vi "MainGUI.vi"() -> ()   [LabVIEW 2018]
uses:
  General/Controls/ScanType.ctl
  General/Controls/Vibratome Parameters.ctl
  General/Controls/Imaging Parameters.ctl
  General/Controls/Scan Direction.ctl
  General/type defines/Alazar parameters.ctl
  Hardware Mfg/AlazarTech SDK/Controls/General Trigger Settings.ctl
  Hardware Mfg/AlazarTech SDK/Controls/Trigger Engine Controls.ctl
  Hardware Mfg/AlazarTech SDK/Controls/Clock Controls.ctl
  Hardware Mfg/AlazarTech SDK/Controls/Alazar Device ID.ctl
  Hardware Mfg/AlazarTech SDK/Controls/Channel Input Controls.ctl
  Hardware Mfg/AlazarTech SDK/Controls/Alazar Acquisition Settings.ctl
  General/Controls/Optical Parameters.ctl
  General/Controls/Translation Stage Parameters.ctl
  Hardware Mfg/Thorlabs Translation Stages/Controls/Translation Stage Cluster.ctl
  General/Controls/Translation Stage Types.ctl
  General/Controls/Go Scan Actions.ctl
  General/Controls/Hardware control.ctl
  General/Controls/Queue Manager Actions.ctl
  General/Controls/MessagePacket.ctl
  General/Controls/QueueNames.ctl
  General/Controls/FGV Actions.ctl
  General/Controls/System Parameters.ctl
  Hardware Mfg/AlazarTech SDK/Controls/Alazar Engine Actions.ctl
  Hardware Mfg/Main Scan Processor Status.vi
  Hardware Mfg/Axsun Laser/Axsun action.ctl
panel:
  in  "Status":string
  in  "Quit":bool
  in  "Acquire":bool
  in  "Control Panel":T1(tab)
  in  "Optical Parameters":T2={"Obj. Focal Length [mm]"=45.0, "Scan Lens EFL[mm]"=59.5, "Tube Lens EFL[mm]"=205.0, "Galvo V Range (+/-)"=10.0, "Galvo Max Half Angle [Deg]"=19.0, "Max Galvo Range[%]"=0.0}
  in  "Galvo HW Parameters":T3={"Analog Out Channel"="GalvoCtrl/ao0,GalvoCtrl/ao1", "Min Voltage"=-10.0, "Max Voltage"=10.0, "Pixel Clock Source"="/GalvoCtrl/PFI0", "Sample Rate"=1000.0, "Line Clock Out Ch"="GalvoCtrl/port0/line0"}
  in  "Imaging Parameter":T4={"Raster Scan Direction"=enum."Uni Directional", "Pixel Dwell Time [Clock Cycles]"=1, "Flyback Time [Clock Cycles]"=200, "XY Center [um]"={"X"=1.0, "Y"=1.0}, "Pixel Step Size [um]"=2.5, "XY Image Size"=enum."2048 x 2048", "Custom"=TRUE, "Custom Size"={"X"=1200, "Y"=1200}, "Line Averages"=1} {"Line Averages" min=1 max=30 step=1; "Flyback Time [Clock Cycles]" max=1000 step=1; "Pixel Step Size [um]" min=0.0 max=10.0 step=0.01; "Custom Size"."Y" min=1 max=30 step=1; "Custom Size"."X" min=1 max=30 step=1; "XY Center [um]"."Y" min=1.0 max=30.0 step=1.0; "XY Center [um]"."X" min=1.0 max=30.0 step=1.0; "Pixel Dwell Time [Clock Cycles]" max=10 step=1}
  in  "Scan Type":T6
  in  "Hardware in":T7
  in  "Alazar parameters":T8={"Trigger Settings"={"General Trigger Settings"={"Trigger Operation"=0, "Coupling ID"=2, "Range ID"=2, "Delay"=0, "Timeout Ticks"=0, "Mode"=1, "Parameter"=1}, "Trigger Engine 1"={"Trigger Engine"=0, "Source"=2, "Slope"=1, "Level"=140}, "Trigger Engine 2"={"Trigger Engine"=1, "Source"=2, "Slope"=1, "Level"=2048}}, "Capture Clock"={"Sample Rate"=100, "Decimation"=0, "Source"=2, "Edge"=0}, "Device ID"={"System ID"=1, "Board ID"=1}, "Ch A Input Control"={"Channel"=1, "Coupling"=2, "Range"=10, "Impedance"=2}, "Ch B Input Control"={"Channel"=2, "Coupling"=2, "Range"=10, "Impedance"=2}, "Acq Settings"={"Window Type"=1, "Record Length"=1440, "Footer"=0, "Offset"=0, "Records Per Buffer"=1220, "Samples per record"=2048, "Records Count (Records/Acq)"=2147483647, "Output Format"=11}} {"Acq Settings"."Output Format" items=["Float Amp"=10, "Float Log"=11, "U16_LOG"=1, "U16_AMP2"=257]; "Acq Settings"."Window Type" items=["DSP_WINDOW_NONE", "DSP_WINDOW_HANNING", "DSP_WINDOW_HAMMING", "DSP_WINDOW_BLACKMAN", "DSP_WINDOW_BLACKMAN_HARRIS", "DSP_WINDOW_BARTLETT"]; "Acq Settings"."Footer" items=["FOOTER_NONE", "FOOTER_NPT"]; "Ch B Input Control"."Channel" items=["A"=1, "B"=2, "C"=4, "D"=8]; "Ch B Input Control"."Coupling" items=["AC"=1, "DC"=2]; "Ch B Input Control"."Range" items=["20 mV"=1, "40 mV"=2, "50 mV"=3, "80 mV"=4, "100 mV"=5, "200 mV"=6, "400 mV"=7, "500 mV"=8, "800 mV"=9, "1 V"=10, "1.25 V"=33, "2 V"=11, "4 V"=12, "5 V"=13, "8 V"=14, "10 V"=15, "20 V"=16]; "Ch B Input Control"."Impedance" items=["1 MOhm"=1, "50 Ohm"=2, ""=0]; "Ch A Input Control"."Channel" items=["A"=1, "B"=2, "C"=4, "D"=8]; "Ch A Input Control"."Coupling" items=["AC"=1, "DC"=2]; "Ch A Input Control"."Range" items=["20 mV"=1, "40 mV"=2, "50 mV"=3, "80 mV"=4, "100 mV"=5, "200 mV"=6, "400 mV"=7, "500 mV"=8, "800 mV"=9, "1 V"=10, "1.25 V"=33, "2 V"=11, "4 V"=12, "5 V"=13, "8 V"=14, "10 V"=15, "20 V"=16]; "Ch A Input Control"."Impedance" items=["1 MOhm"=1, "50 Ohm"=2, ""=0]; "Capture Clock"."Edge" items=["Rising", "Falling"]; "Capture Clock"."Source" items=["Internal"=1, "Fast External"=2, "Medium External"=3, "Slow External"=4, "External AC"=5, "External DC"=6, "External 10MHz"=7]; "Trigger Settings"."General Trigger Settings"."Trigger Operation" items=["J", "K", "J OR K", "J AND K", "J XOR K", "J AND NOT K", "NOT J AND K"]; "Trigger Settings"."General Trigger Settings"."Coupling ID" items=["AC"=1, "DC"=2]; "Trigger Settings"."General Trigger Settings"."Range ID" items=["5 V", "1 V", "TTL"]; "Trigger Settings"."Trigger Engine 1"."Trigger Engine" items=["J", "K"]; "Trigger Settings"."Trigger Engine 1"."Source" items=["A", "B", "External", "Disable", "C", "D"]; "Trigger Settings"."Trigger Engine 1"."Slope" items=["Positive"=1, "Negative"=2]; "Trigger Settings"."Trigger Engine 2"."Trigger Engine" items=["J", "K"]; "Trigger Settings"."Trigger Engine 2"."Source" items=["A", "B", "External", "Disable", "C", "D"]; "Trigger Settings"."Trigger Engine 2"."Slope" items=["Positive"=1, "Negative"=2]}
  in  "Vibratome":T15={"Z Bottom [mm]"=0.0, "Pre Cut Dwell [s]"=0.0, "Blade Frequency [RPM]"=0, "Slice Speed [mm/s]"=0.0, "Post Cut Dwell [s]"=0.0, "Ramp Time [s]"=0.0, "Start X [mm]"=0.0, "Start Y [mm]"=0.0, "Slice Length [mm]"=0.0, "Slice Axis"=enum."X Axis", "Controller VISA Ref"="COM4"}
  in  "Mosaic Paramter":T16
  in  "#pixels to save":u32=70
  in  "Start pixel for save":u32=70
  in  "Save?":bool
  in  "Center Galvos":bool
  in  "path":path=path "C:/Users/BOAS-USER/Documents/Data/0520/test"
  in  "#pixels to display":i32=500
  in  "Channel":u32(ring)=1 items=["A"=1, "B"=2, "A + B"=3, "C"=4, "A + C"=5, "A + B"=6, "D"=8, "A + D"=9, "B + D"=10, "C + D"=12, "A + B + C + D"=15]
  out "#C-lines":i32=1
  in  "Start pixel for display":i32=1
  out "Current Position":cluster{"X":dbl, "Y":dbl}
  out "Current state":T17
  in  "Table Stages":T18={"X Stage"={"Position"=0.0, "Is.Enabled?"=FALSE, "Is.Connected?"=FALSE, "Device SN"="45876539", "AccelerationMaximum"=20.0, "VelocityMaximum"=20.0, "Acceleration"=10.0, "Velocity"=10.0, "waitTimeout (ms)"=1000, "Model"=enum."Thorlabs LTS", "Is.Homed?"=FALSE}, "Y Stage"={"Position"=0.0, "Is.Enabled?"=FALSE, "Is.Connected?"=FALSE, "Device SN"="45875512", "AccelerationMaximum"=20.0, "VelocityMaximum"=20.0, "Acceleration"=10.0, "Velocity"=10.0, "waitTimeout (ms)"=1000, "Model"=enum."Thorlabs LTS", "Is.Homed?"=FALSE}, "Z Stage"={"Position"=0.0, "Is.Enabled?"=FALSE, "Is.Connected?"=FALSE, "Device SN"="49876924", "AccelerationMaximum"=8.0, "VelocityMaximum"=3.0, "Acceleration"=4.0, "Velocity"=2.0, "waitTimeout (ms)"=1000, "Model"=enum."Thorlabs MLJ", "Is.Homed?"=FALSE}}
  out "Image":T21(plugin-control)
  out "Control Class ID":u32[](array[numeric])
  out "Label Name":string[][](array[string])
  # "Image Settings"
  # "Optical Settings"
  # "X"
  # "X"
  # "Vibratome Settings"
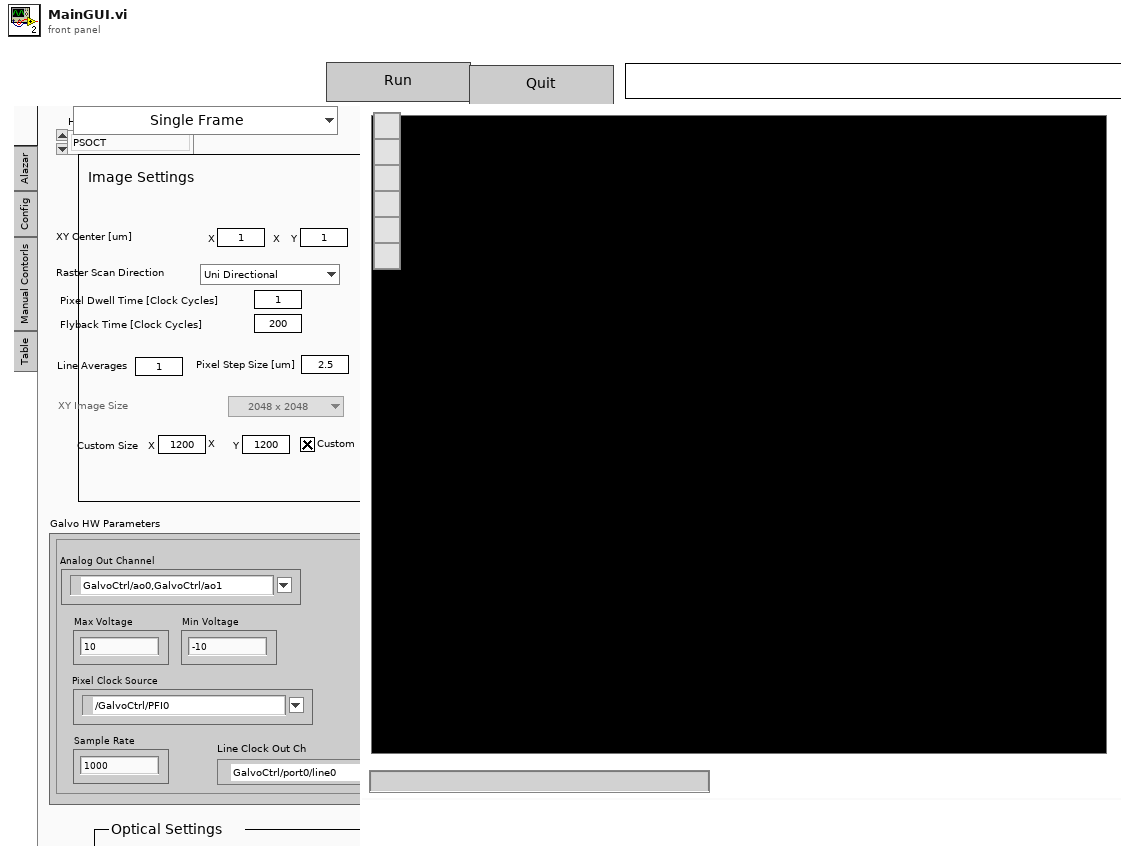
[diagram p1: front panel]
types:
  T1 = enum32{"Galvo", "Alazar", "Config", "Manual Contorls", "Table"}
  T2 = typedef "Optical Parameters.ctl" = cluster{"Obj. Focal Length [mm]":dbl, "Scan Lens EFL[mm]":dbl, "Tube Lens EFL[mm]":dbl, "Galvo V Range (+/-)":dbl, "Galvo Max Half Angle [Deg]":dbl, "Max Galvo Range[%]":dbl}
  T3 = cluster{"Analog Out Channel":tag, "Min Voltage":dbl, "Max Voltage":dbl, "Pixel Clock Source":tag, "Sample Rate":dbl, "Line Clock Out Ch":tag}
  T4 = typedef "Imaging Parameters.ctl" = cluster{"Raster Scan Direction":T5, "Pixel Dwell Time [Clock Cycles]":u16, "Flyback Time [Clock Cycles]":u16, "XY Center [um]":cluster{"X":dbl, "Y":dbl}, "Pixel Step Size [um]":dbl, "XY Image Size":enum16{"32 x 32", "64 x 64", "128 x 128", "256 x 256", "512 x 512", "1024 x 1024", "2048 x 2048"}, "Custom":bool, "Custom Size":cluster{"X":u16, "Y":u16}, "Line Averages":u8}
  T5 = typedef "Scan Direction.ctl" = enum16{"Uni Directional", "Bi Directional", "None"}
  T6 = typedef "ScanType.ctl" = enum16{"Single Frame", "Continuous Frame", "ROI Line", "Vibratome", "Mosaic", "Mosaic + Slice"}
  T7 = typedef "Hardware control.ctl" = enum16{"PSOCT", "Thorlabs OCT"}
  T8 = typedef "Alazar parameters.ctl" = cluster{"Trigger Settings":cluster{"General Trigger Settings":T9, "Trigger Engine 1":T10, "Trigger Engine 2":T10}, "Capture Clock":T11, "Device ID":T12, "Ch A Input Control":T13, "Ch B Input Control":T13, "Acq Settings":T14}
  T9 = typedef "General Trigger Settings.ctl" = cluster{"Trigger Operation":u32, "Coupling ID":u32, "Range ID":u32, "Delay":u32, "Timeout Ticks":u32, "Mode":u32, "Parameter":u32}
  T10 = typedef "Trigger Engine Controls.ctl" = cluster{"Trigger Engine":u32, "Source":u32, "Slope":u32, "Level":u32}
  T11 = typedef "Clock Controls.ctl" = cluster{"Sample Rate":u32, "Decimation":u32, "Source":u32, "Edge":u32}
  T12 = typedef "Alazar Device ID.ctl" = cluster{"System ID":u32, "Board ID":u32}
  T13 = typedef "Channel Input Controls.ctl" = cluster{"Channel":u8, "Coupling":u32, "Range":u32, "Impedance":u32}
  T14 = typedef "Alazar Acquisition Settings.ctl" = cluster{"Window Type":u32, "Record Length":u32, "Footer":u32, "Offset":u32, "Records Per Buffer":u32, "Samples per record":u32, "Records Count (Records/Acq)":u32, "Output Format":u32}
  T15 = typedef "Vibratome Parameters.ctl" = cluster{"Z Bottom [mm]":dbl, "Pre Cut Dwell [s]":dbl, "Blade Frequency [RPM]":u16, "Slice Speed [mm/s]":dbl, "Post Cut Dwell [s]":dbl, "Ramp Time [s]":dbl, "Start X [mm]":dbl, "Start Y [mm]":dbl, "Slice Length [mm]":dbl, "Slice Axis":enum16{"X Axis", "Y Axis", "Z Axis"}, "Controller VISA Ref":refnum<visa-resource-name>}
  T16 = cluster{"X Axis":cluster{"Start [mm]":dbl, "FOV[mm]":dbl, "End [mm]":dbl}, "Y Axis":cluster{"Start [mm]":dbl, "FOV[mm]":dbl, "End [mm]":dbl}, "Scan Pattern":enum16{"Uni-directional", "Bi-Directional", "Spiral Out", "Spiral In"}, "Overlap Options":cluster{"Overlap Type":enum16{"No Overlap", "X Only", "Y Only", "X and Y"}, "Percent Overlap":u8, "Justify":enum16{"Start", "Center", "End"}}}
  T17 = typedef "Go Scan Actions.ctl" = enum16{"Init", "Ready for acquire", "Init Scan Head", "Init Table Stage", "Init Vibratome", "Generate Mosaic", "Export info", "Go Image Home", "Go Mosaic", "Acquire Image", "Go Vibratome", "Slice", "Finished"}
  T18 = typedef "Translation Stage Parameters.ctl" = cluster{"X Stage":T19, "Y Stage":T19, "Z Stage":T19}
  T19 = typedef "Translation Stage Cluster.ctl" = cluster{"Position":dbl, "Is.Enabled?":bool, "Is.Connected?":bool, "Device SN":string, "AccelerationMaximum":dbl, "VelocityMaximum":dbl, "Acceleration":dbl, "Velocity":dbl, "waitTimeout (ms)":i32, "Model":T20, "Is.Homed?":bool}
  T20 = typedef "Translation Stage Types.ctl" = enum16{"None", "Thorlabs LTS", "Thorlabs MLJ"}
  T21 = typedef "IMAQ Image.ctl" = refnum<image>
  T22 = typedef "QueueNames.ctl" = enum16{"Main GUI", "Main Scan Processor", "Main Processing", "Main Saving", "Main Display", "Main Table Stage GUI", "Main Table Stage Proc.", "Scan Engine", "Vibratome GUI", "Vibratome Processor", "Slice Engine"}
  T23 = typedef "Queue Manager Actions.ctl" = enum16{"Init", "Enqueue", "Enqueue All", "Preview Queue", "Dequeue", "Get Status", "Flush Queue", "Flush All Queues", "Release All Queues", "Release Queue", "Enqueue at Opposite End"}
  T24 = typedef "MessagePacket.ctl" = cluster{"Message":string, "Parameter":variant}
  T25 = typedef "FGV Actions.ctl" = enum16{"Init", "Set", "Get", "Clear"}
  T26 = typedef "System Parameters.ctl" = cluster{"Optical Parameters":T2, "Vibratome":T15, "Table Stages":T18, "Imaging Parameter":T4, "Galvo HW Parameters":cluster{"Analog Out Channel":tag, "Min Voltage":dbl, "Max Voltage":dbl, "Pixel Clock Source":tag, "Sample Rate":dbl, "Line Clock Out Ch":tag}, "Alazar parameters":T8, "Mosaic Paramter":cluster{"X Axis":cluster{"Start [mm]":dbl, "Steps [pts]":u16, "End [mm]":dbl}, "Y Axis":cluster{"Start [mm]":dbl, "Steps [pts]":u16, "End [mm]":dbl}, "Scan Pattern":enum16{"Uni-directional", "Bi-Directional", "Spiral Out", "Spiral In"}, "Overlap Options":cluster{"Overlap Type":enum16{"No Overlap", "X Only", "Y Only", "X and Y"}, "Percent Overlap":u8, "Justify":enum16{"Start", "Center", "End"}}}}
  T27 = typedef "Axsun action.ctl" = enum16{"GetSystemStatus", "Clock delay", "GetLaserOnTime", "GetWaveLengthAtSweptTrigger", "Source current ON", "GetSerialNum", "GetControlVersion", "Laser ON", "Laser OFF", "Source current OFF", "Get laser handle", "Start Network Control Interface", "stop", "Create handle"}
  T28 = typedef "Alazar Engine Actions.ctl" = enum16{"Init", "Config Clock", "Config Ch", "Config Trig", "Config Non-FFT Acq.", "Non-FFT Acquire", "Load background from Non-FFT buffer", "enable background subtrac", "disable background subtrac", "load background from file", "load background from elsewhere", "start acquire", "background subtraction", "Config Acq.", "Acquire", "UnInit"}
  T29 = enum16{"Set Configuration", "Get Configuration", "Enable Motor", "Disable Motor", "Get Status", "Open Session", "Close Session", "Set Limits", "Get Limits"}
  T30 = typedef "Image Type" = u32
  T31 = enum16{"32 x 32", "64 x 64", "128 x 128", "256 x 256", "512 x 512", "1024 x 1024", "2048 x 2048"}
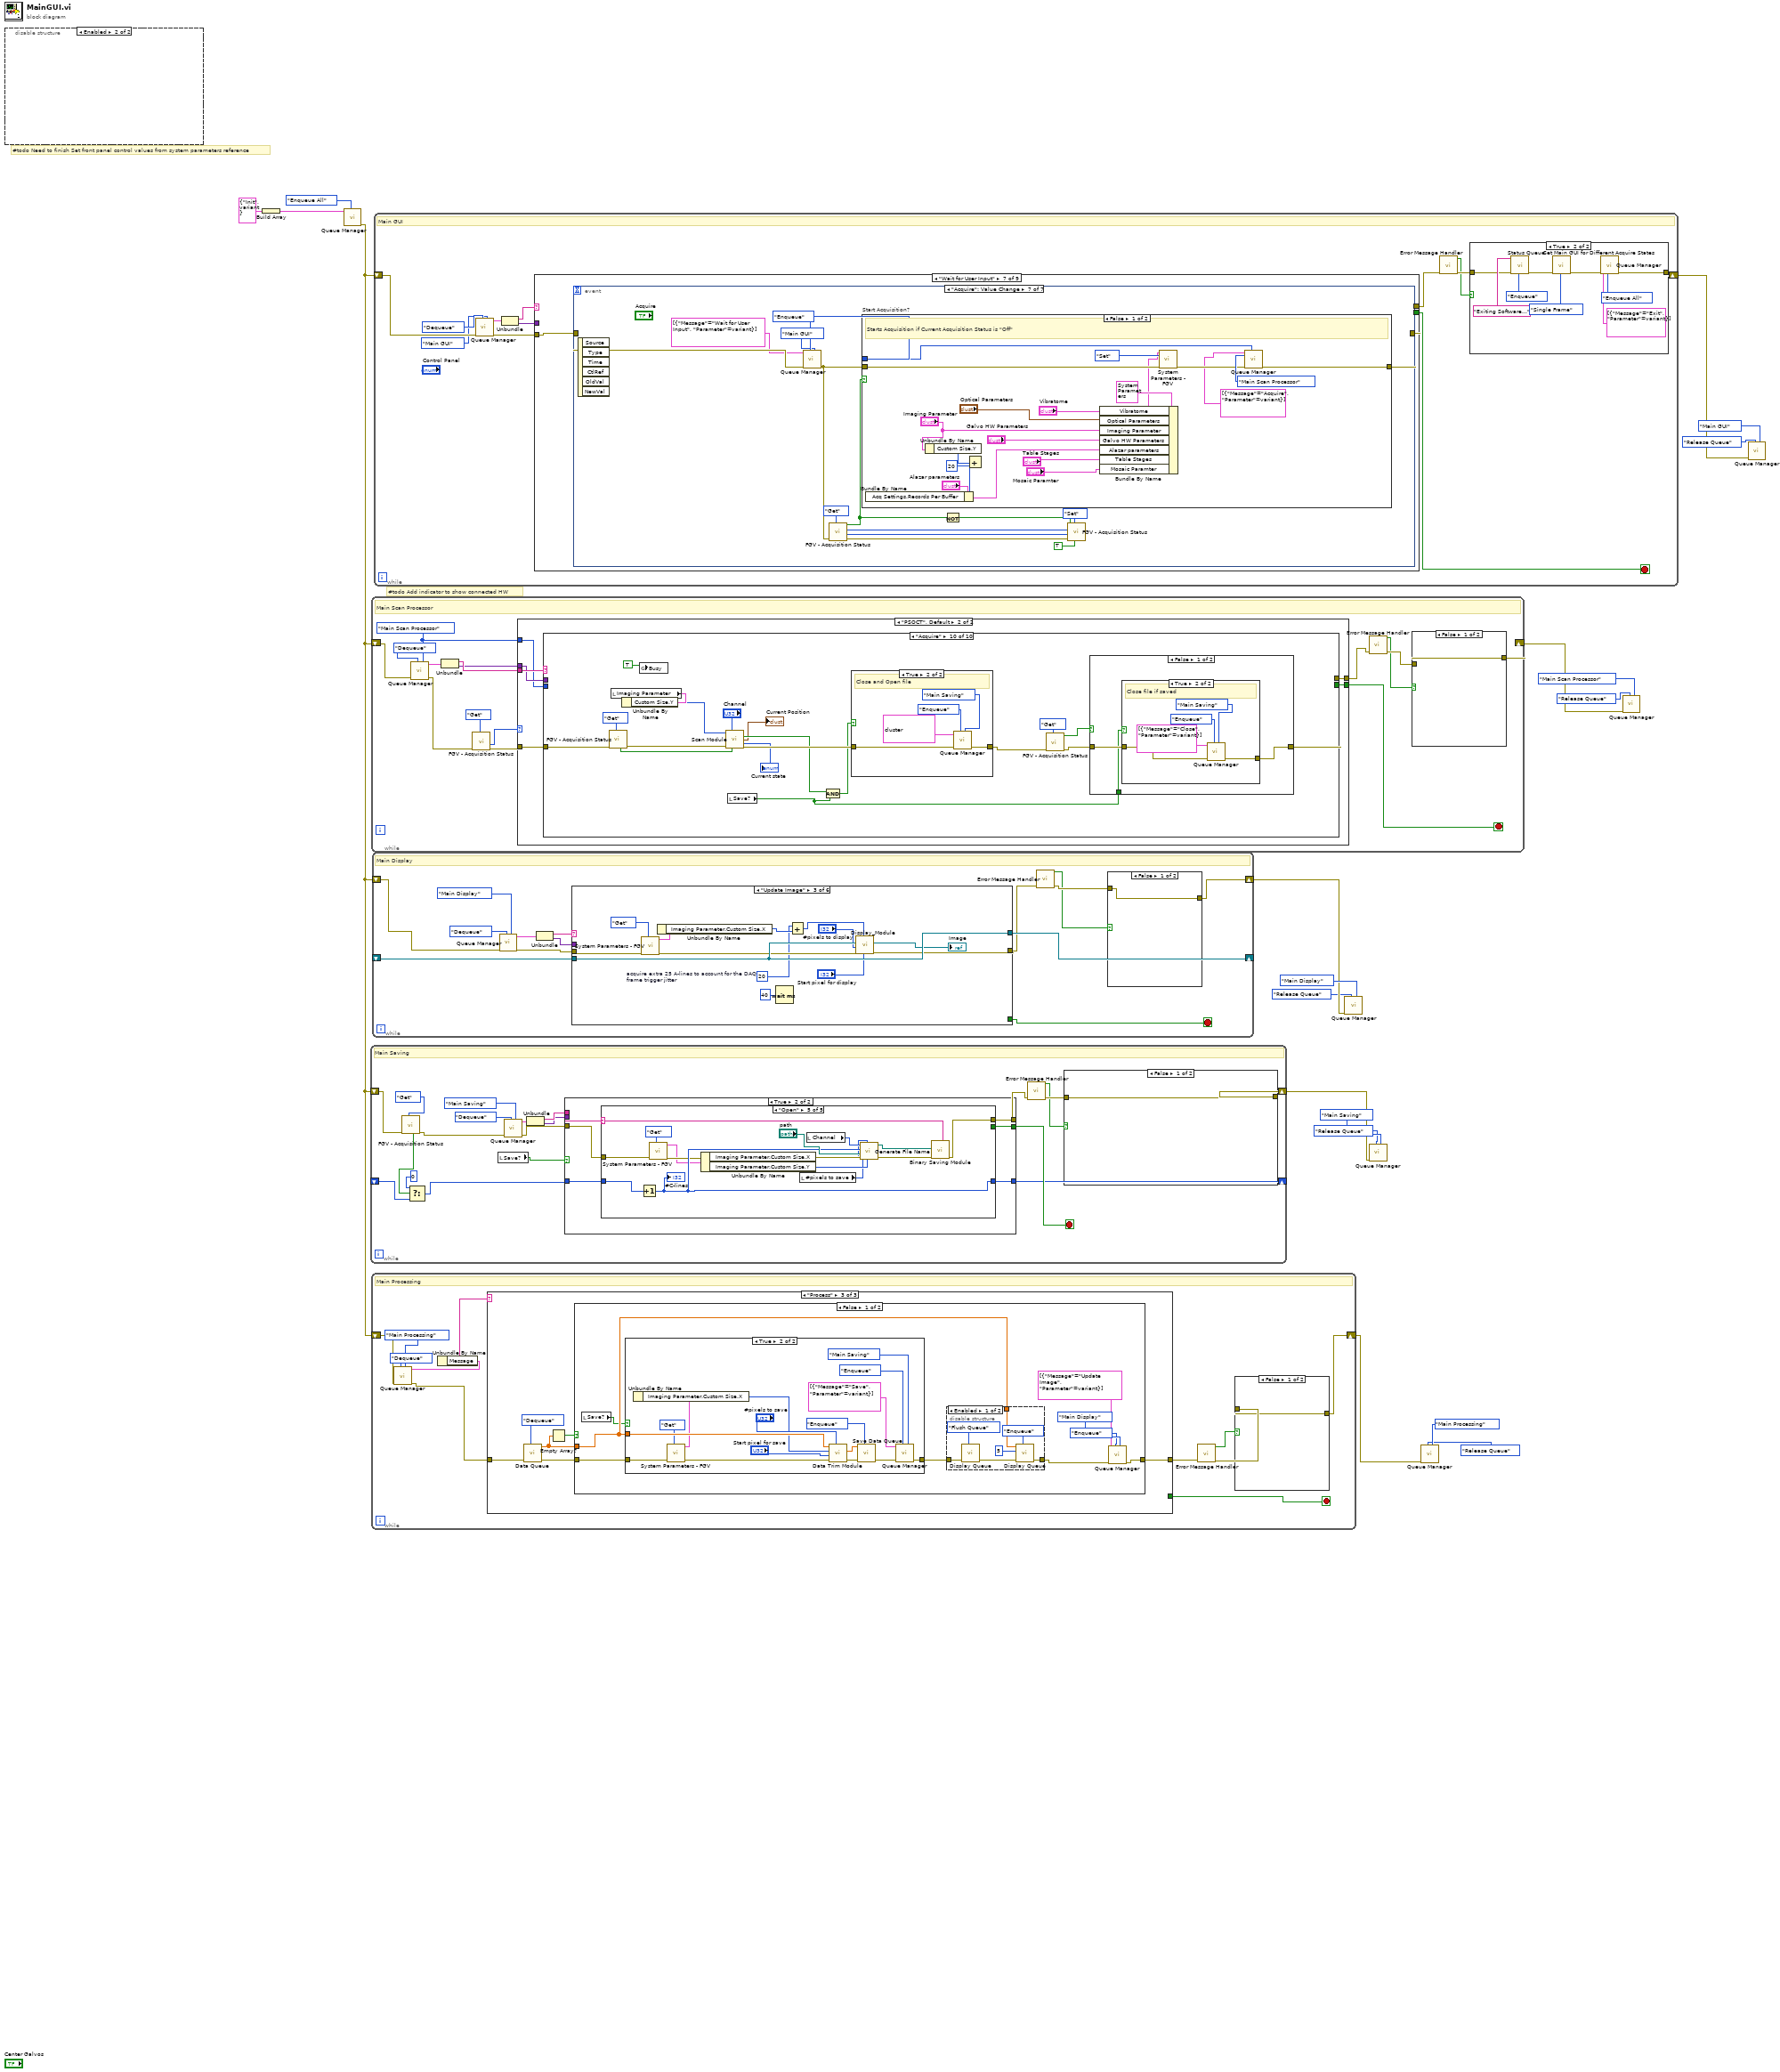
[diagram p0: block diagram]
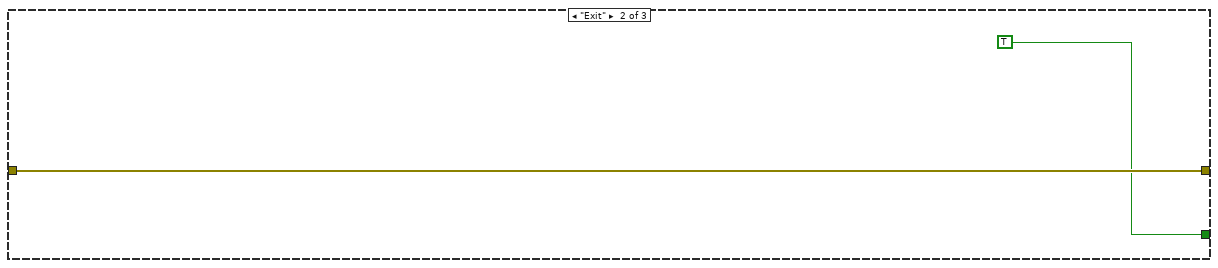
[diagram p3: hidden frame]
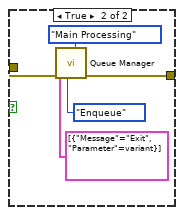
[diagram p7: hidden frame]
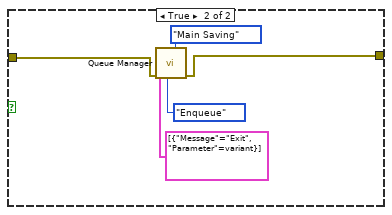
[diagram p8: hidden frame]
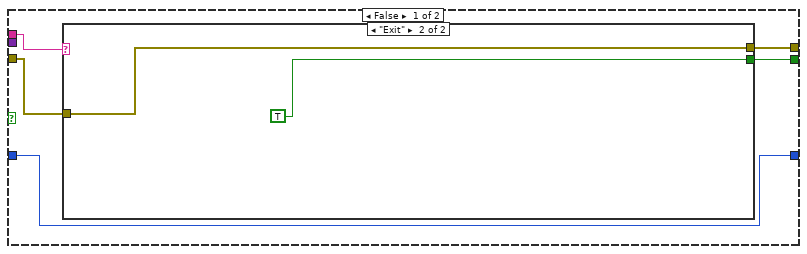
[diagram p9: hidden frame]
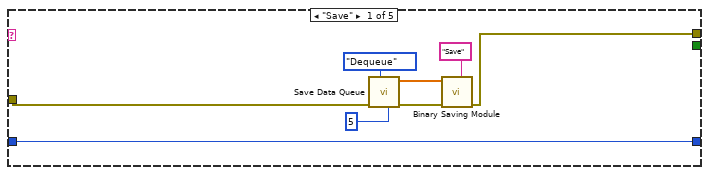
[diagram p11: hidden frame]
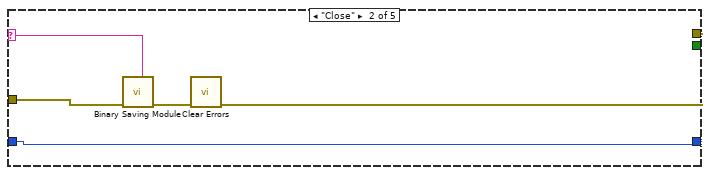
[diagram p12: hidden frame]
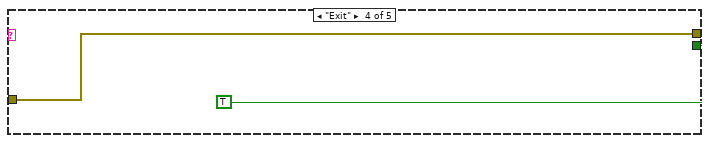
[diagram p14: hidden frame]
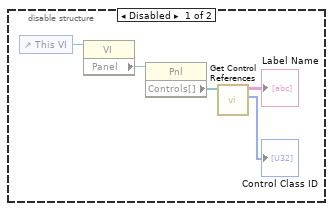
[diagram p15: hidden frame]
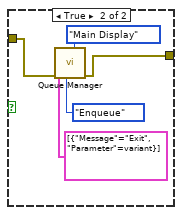
[diagram p16: hidden frame]
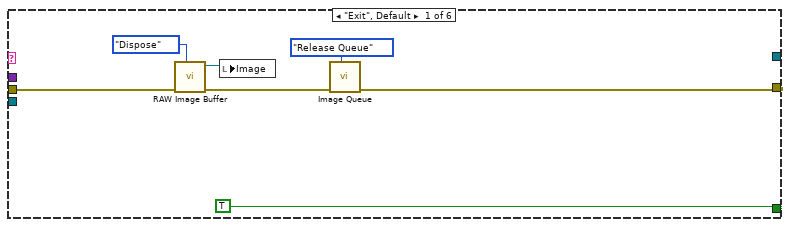
[diagram p17: hidden frame]
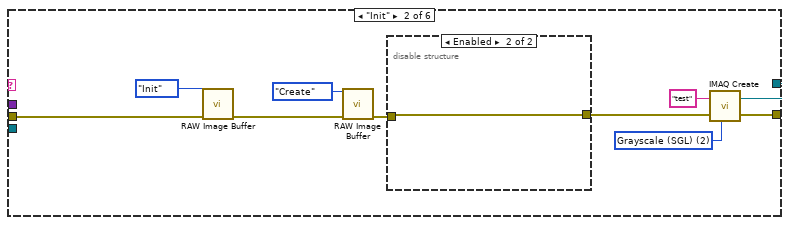
[diagram p18: hidden frame]
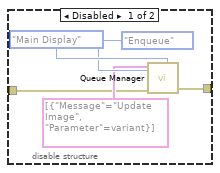
[diagram p19: hidden frame]
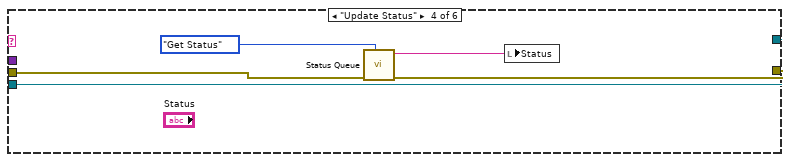
[diagram p20: hidden frame]
diagram:
  # "#todo Add indicator to show connected HW"
  # "#todo Need to finish Set front panel control values from system parameters reference"
  n1 = disable-structure shown="Enabled" {
    frame Disabled {
      n2 = control-ref of="This VI"() -> (w24:refnum<vi>)
      n3 = property class="VI"(reference=w24) -> ("Panel"=w23:refnum<vi>)  [unwired: 1 in, 2 out]
      n4 = property class="Pnl"(reference=w23) -> ("Controls[]"=w22:refnum<vi>[])  [unwired: 1 in, 2 out]
      n5 = call "Get Control References.vi"("Control References"=w22) -> ("Control Class ID"=→"Control Class ID":u32[], "Label Name"=→"Label Name":string[][])  [unwired: 8 in, 1 out]
    }
    frame Enabled {
    }
  }
  n6 = Build Array(T24 {"Message"="Init", "Parameter"=variant} ("Message Packet [In]")) -> (w17:T24[])
  n7 = call "Queue Manager.vi"("Action"=Queue_Manager_Actions."Enqueue All", "Message Packet Array"=w17) -> ("Error Out"=w1:errorcluster)  [unwired: 5 in, 4 out]
  n8 = while {
    shift-right: [w31] -> w5
    shift-left: w1 -> [w28]
    shift-right: [w43] -> _
    shift-left: _ -> [w41]
    stop <- w44 stop-if-true
    # "Main Saving"
    n9 = call "FGV - Acquisition Status.vi"("Actions"=FGV_Actions."Get", "Error In"=w28) -> ("Error Out"=w27:errorcluster, "Edge Status Out"=w25:bool)  [unwired: 5 in, 3 out]
    n10 = Select(t=u32 0, s=w25, f=w41) -> (s? t:f=w40:u32)
    n11 = local read "Save?"() -> (w29:bool)
    n12 = call "Queue Manager.vi"("Queue Name"=QueueNames."Main Saving", "Action"=Queue_Manager_Actions."Dequeue", "Error In"=w27) -> ("Error Out"=w34:errorcluster, "Message Packet [Out]"=w39:T24)  [unwired: 4 in, 3 out]
    n13 = Unbundle(w39) -> ("Message"=w36:string, "Parameter"=w35:variant)
    n14 = case shown="True" w29 {
      tunnel: [w54 w64] -> w33
      tunnel: [w51 w63] -> w44
      tunnel: [w52 w62] -> w43
      tunnel: w40 -> [w52 w61]
      tunnel: w36 -> [w53 w60]
      tunnel: w35 -> [_ _]
      tunnel: w34 -> [w55 w59]
      frame False {
        n15 = case shown="\"Exit\"" w53 {
          tunnel: [w56 w57] -> w54
          tunnel: w55 -> [w56 w57]
          tunnel: [_ TRUE] -> w51
          frame "Init", Default {
          }
          frame "Exit" {
          }
        }
      }
      frame True {
        n16 = case shown="\"Open\"" w60 {
          selector: w60 -> [_ w76 _ _ w95]
          tunnel: [w70 w73 w79 w80 w93] -> w64
          tunnel: w59 -> [w72 w77 w79 w80 w87]
          tunnel: [_ _ _ TRUE _] -> w63
          tunnel: [w71 w74 w78 _ w90] -> w62
          tunnel: w61 -> [w71 w74 w78 _ w89]
          frame "Save" {
            n17 = call "Save Data Queue.vi"("timeout in ms (-1)"=5, "Action"=Queue_Manager_Actions."Dequeue", "error in (no error)"=w72) -> ("error out"=w68:errorcluster, "data out"=w69:sgl[])  [unwired: 5 in, 2 out]
            n18 = call "Binary Saving Module.vi"("action"="Save", "error in"=w68, "data in"=w69) -> ("error out"=w70:errorcluster)  [unwired: 8 in]
          }
          frame "Close" {
            n19 = call "Binary Saving Module.vi"("action"=w76, "error in"=w77) -> ("error out"=w75:errorcluster)  [unwired: 9 in]
            n20 = call <vilib>:"Clear Errors.vi"("error in (no error)"=w75) -> ("error out"=w73:errorcluster)  [unwired: 5 in, 1 out]
          }
          frame "Init", Default {
          }
          frame "Exit" {
          }
          frame "Open" {
            n21 = Increment(x=w89) -> (x+1=w90:u32)
            "#C-lines" <- w90
            n22 = call "System Parameters - FGV.vi"("Actions"=FGV_Actions."Get", "Error In"=w87) -> ("Error Out"=w88:errorcluster, "System Parameters"=w85:T26)  [unwired: 8 in]
            n23 = Unbundle By Name(w85) -> ("Imaging Parameter.Custom Size.X"=w84:u16, "Imaging Parameter.Custom Size.Y"=w83:u16)
            n24 = local read "#pixels to save"() -> (w82:u32)
            n25 = local read "Channel"() -> (w91:u32)
            n26 = call "Generate File Name.vi"("Y"=w83, "X"=w84, "Z"=w82, "path"="path", "#C scan"=w90, "Channel"=w91) -> ("appended path"=w94:path)  [unwired: 5 in]
            n27 = call "Binary Saving Module.vi"("action"=w95, "error in"=w88, "file path (use dialog)"=w94) -> ("error out"=w93:errorcluster)  [unwired: 8 in]
          }
        }
      }
    }
    n28 = call "Error Message Handler.vi"("Error In"=w33) -> ("Error Out"=w32:errorcluster, "T button?"=w30:bool)  [unwired: 9 in]
    n29 = case shown="False" w30 {
      tunnel: [w45 w48] -> w31
      tunnel: w32 -> [w45 w46]
      frame False {
      }
      frame True {
        n30 = call "Queue Manager.vi"("Queue Name"=QueueNames."Main Saving", "Action"=Queue_Manager_Actions."Enqueue", "Error In"=w46, "Message Packet Array"=T24[] [{"Message"="Exit", "Parameter"=variant}] ("Message Packet [In]")) -> ("Error Out"=w48:errorcluster)  [unwired: 3 in, 4 out]
      }
    }
  }
  n31 = while {
    shift-right: [w100] -> w11
    shift-left: w1 -> [w109]
    stop <- w110 stop-if-true
    w104 = QueueNames."Main Scan Processor" ("Queue Name")
    # "Main Scan Processor"
    n32 = call "Queue Manager.vi"("Queue Name"=w104, "Action"=Queue_Manager_Actions."Dequeue", "Error In"=w109) -> ("Error Out"=w99:errorcluster, "Message Packet [Out]"=w107:T24)  [unwired: 4 in, 3 out]
    n33 = Unbundle(w107) -> ("Message"=w106:string, "Parameter"=w105:variant)
    n34 = call "FGV - Acquisition Status.vi"("Actions"=FGV_Actions."Get", "Error In"=w99) -> ("Error Out"=w98:errorcluster, "Hardware out"=w96:T7)  [unwired: 5 in, 3 out]
    n35 = case shown="\"PSOCT\", Default" w96 {
      tunnel: [w111 w125] -> w110
      tunnel: w106 -> [w114 w124]
      tunnel: w105 -> [_ w123]
      tunnel: w104 -> [_ w122]
      tunnel: w98 -> [w113 w121]
      tunnel: [w112 w120] -> w103
      frame "Thorlabs OCT" {
        n36 = case shown="\"Acquire\"" w114 {
          tunnel: w113 -> [w115 w117 w119]
          tunnel: [w115 w116 w119] -> w112
          tunnel: [_ _ TRUE] -> w111
          frame "False", Default {
          }
          frame "Acquire" {
            n37 = call "Scan Module.vi"("Error In"=w117) -> ("Error Out"=w116:errorcluster)  [unwired: 10 in, 4 out]
          }
          frame "Exit" {
          }
        }
      }
      frame "PSOCT", Default {
        n38 = case shown="\"Acquire\"" w124 {
          tunnel: w123 -> [_ _ _ _ _ _ _ _ _ _]
          tunnel: [w126 w128 w134 w135 w137 w139 w159 w170 w180 w195] -> w120
          tunnel: [TRUE _ _ _ _ _ _ _ _ _] -> w125
          tunnel: w122 -> [_ _ w133 _ _ _ _ _ _ _]
          tunnel: w121 -> [w126 w128 w129 w135 w137 w138 w154 w169 w180 w185]
          frame "Exit" {
          }
          frame "Init" {
          }
          frame "Init Hardware" {
            n39 = global write "Main Scan Processor Status.vi" "Busy"(TRUE ("Busy")) -> ()
            n40 = call "Queue Manager.vi"("Queue Name"=w133, "Action"=Queue_Manager_Actions."Enqueue", "Error In"=w129, "Message Packet Array"=T24[] [{"Message"="Init Table Stages", "Parameter"=variant}, {"Message"="Init DAQ", "Parameter"=variant}, {"Message"="Init Vibratome", "Parameter"=variant}, {"Message"="Init Laser", "Parameter"=variant}, {"Message"="Init Alazar", "Parameter"=variant}, {"Message"="", "Parameter"=variant}, {"Message"="", "Parameter"=variant}]) -> ("Error Out"=w134:errorcluster)  [unwired: 3 in, 4 out]
          }
          frame "Init Table Stages" {
            n41 = global write "Main Scan Processor Status.vi" "Busy"(TRUE ("Busy")) -> ()
          }
          frame "Init DAQ" {
          }
          frame "Init Laser" {
            n42 = disable-structure shown="Disabled" {
              disable-tunnel: w138 -> [w141 _]
              disable-tunnel: [w140 _] -> w139
              frame Disabled {
                n43 = call "Axsun module.vi"("Action"=Axsun_action."Create handle", "error in (no error)"=w141) -> ("error out"=w151:errorcluster)  [unwired: 8 in, 1 out]
                n44 = call "Axsun module.vi"("Action"=Axsun_action."GetControlVersion", "error in (no error)"=w151) -> ("error out"=w150:errorcluster)  [unwired: 8 in, 1 out]
                n45 = call "Axsun module.vi"("Action"=Axsun_action."Start Network Control Interface", "error in (no error)"=w150) -> ("error out"=w149:errorcluster)  [unwired: 8 in, 1 out]
                n46 = call "Axsun module.vi"("Action"=Axsun_action."Get laser handle", "error in (no error)"=w149) -> ("error out"=w148:errorcluster)  [unwired: 8 in, 1 out]
                n47 = call "Axsun module.vi"("Action"=Axsun_action."GetSerialNum", "error in (no error)"=w148) -> ("error out"=w147:errorcluster)  [unwired: 8 in, 1 out]
                n48 = call "Axsun module.vi"("Action"=Axsun_action."GetSystemStatus", "error in (no error)"=w147) -> ("error out"=w140:errorcluster)  [unwired: 8 in, 1 out]
              }
              frame Enabled {
              }
            }
          }
          frame "Init Alazar" {
            n49 = call "System Parameters - FGV.vi"("Actions"=FGV_Actions."Get", "Error In"=w154) -> ("Error Out"=w157:errorcluster, "System Parameters"=w156:T26)  [unwired: 8 in]
            n50 = Unbundle By Name(w156) -> ("Alazar parameters"=w155:T8)
            n51 = Unbundle By Name(w155) -> ("Device ID"=w160:T12)
            n52 = case shown="16" 32 {
              tunnel: w160 -> [w163 w167]
              tunnel: [w162 w166] -> w159
              tunnel: w157 -> [w164 w165]
              frame 0, Default {
                n53 = call "AlazarEngine.vi"("Action"=Alazar_Engine_Actions."Init", "error in (no error)"=w164, "Device ID"=w163) -> ("error out"=w162:errorcluster)  [unwired: 6 in, 2 out]
              }
              frame 16 {
                n54 = call "Alazar module U16.vi"("Action"=Alazar_Engine_Actions."Init", "error in (no error)"=w165, "Device ID"=w167) -> ("error out"=w166:errorcluster)  [unwired: 6 in, 2 out]
              }
            }
          }
          frame "Init Vibratome" {
            n55 = disable-structure shown="Disabled" {
              disable-tunnel: w169 -> [w176 _]
              disable-tunnel: [w175 _] -> w170
              frame Disabled {
                n56 = call "System Parameters - FGV.vi"("Actions"=FGV_Actions."Get") -> ("System Parameters"=w173:T26)  [unwired: 9 in, 1 out]
                n57 = Unbundle By Name(w173) -> ("Vibratome.Controller VISA Ref"=w172:refnum<visa-resource-name>)
                n58 = call "MCDC3006 Module.vi"("Actions"=T29."Open Session", "Error In"=w176, "VISA resource name"=w172) -> ("Error Out"=w178:errorcluster)  [unwired: 4 in, 4 out]
                n59 = call "MCDC3006 Module.vi"("Actions"=T29."Enable Motor", "Error In"=w178) -> ("Error Out"=w175:errorcluster)  [unwired: 5 in, 4 out]
              }
              frame Enabled {
              }
            }
            n60 = global write "Main Scan Processor Status.vi" "Busy"(TRUE ("Busy")) -> ()
          }
          frame "Idle", Default {
            n61 = global write "Main Scan Processor Status.vi" "Busy"(FALSE ("Busy")) -> ()
          }
          frame "Acquire" {
            n62 = call "FGV - Acquisition Status.vi"("Actions"=FGV_Actions."Get", "Error In"=w185) -> ("Error Out"=w184:errorcluster, "Edge Status Out"=w182:bool)  [unwired: 5 in, 3 out]
            n63 = local read "Imaging Parameter"() -> (w190:T4)
            n64 = Unbundle By Name(w190) -> ("Custom Size.Y"=w189:u16)
            n65 = global write "Main Scan Processor Status.vi" "Busy"(TRUE ("Busy")) -> ()
            n66 = call "Scan Module.vi"("#B scans"=w189, "Channel"="Channel", "Error In"=w184, "Start Acquire?"=w182) -> ("Ready for next C-scan?"=w197:bool, "Current Position"=→"Current Position":cluster{"X":dbl, "Y":dbl}, "Current state"=→"Current state":T17, "Error Out"=w198:errorcluster)  [unwired: 7 in, 1 out]
            n67 = local read "Save?"() -> (w186:bool)
            n68 = And(x=w197, y=w186) -> (x .and. y?=w196:bool)
            n69 = case shown="True" w196 {
              tunnel: w198 -> [w215 w218]
              tunnel: [w215 w217] -> w193
              frame False {
              }
              frame True {
                # "Close and Open file"
                n70 = call "Queue Manager.vi"("Queue Name"=QueueNames."Main Saving", "Action"=Queue_Manager_Actions."Enqueue", "Error In"=w218, "Message Packet Array"=T24[] [{"Message"="Close", "Parameter"=variant}, {"Message"="Open", "Parameter"=variant}] ("Message Packet [In]")) -> ("Error Out"=w217:errorcluster)  [unwired: 3 in, 4 out]
              }
            }
            n71 = call "FGV - Acquisition Status.vi"("Actions"=FGV_Actions."Get", "Error In"=w193) -> ("Error Out"=w192:errorcluster, "Level Status Out"=w191:bool)  [unwired: 5 in, 3 out]
            n72 = case shown="False" w191 {
              tunnel: w192 -> [w203 w212]
              tunnel: [w202 w211] -> w195
              tunnel: w186 -> [w201 _]
              frame False {
                n73 = case shown="True" w201 {
                  tunnel: w203 -> [w204 w207]
                  tunnel: [w204 w206] -> w202
                  frame False {
                    # "Close file if saved"
                  }
                  frame True {
                    # "Close file if saved"
                    n74 = call "Queue Manager.vi"("Queue Name"=QueueNames."Main Saving", "Action"=Queue_Manager_Actions."Enqueue", "Error In"=w207, "Message Packet Array"=T24[] [{"Message"="Close", "Parameter"=variant}] ("Message Packet [In]")) -> ("Error Out"=w206:errorcluster)  [unwired: 3 in, 4 out]
                  }
                }
              }
              frame True {
                # "Continue acquire if not finished"
                n75 = call "Queue Manager.vi"("Queue Name"=QueueNames."Main Scan Processor", "Action"=Queue_Manager_Actions."Enqueue", "Error In"=w212, "Message Packet Array"=T24[] [{"Message"="Acquire", "Parameter"=variant}] ("Message Packet [In]")) -> ("Error Out"=w211:errorcluster)  [unwired: 3 in, 4 out]
              }
            }
          }
        }
      }
    }
    n76 = call "Error Message Handler.vi"("Error In"=w103) -> ("Error Out"=w102:errorcluster, "T button?"=w101:bool)  [unwired: 9 in]
    n77 = case shown="False" w101 {
      tunnel: w102 -> [w221 w223]
      tunnel: [w221 w224] -> w100
      frame False {
      }
      frame True {
        n78 = call "Queue Manager.vi"("Queue Name"=QueueNames."Main Scan Processor", "Action"=Queue_Manager_Actions."Enqueue", "Error In"=w223, "Message Packet Array"=T24[] [{"Message"="Exit", "Parameter"=variant}] ("Message Packet [In]")) -> ("Error Out"=w224:errorcluster)  [unwired: 3 in, 4 out]
      }
    }
  }
  n79 = while "Main Data Processing" {
    shift-right: [w233] -> w2
    shift-left: w1 -> [w237]
    stop <- w227 stop-if-true
    # "Main Processing"
    n80 = call "Queue Manager.vi"("Queue Name"=QueueNames."Main Processing", "Action"=Queue_Manager_Actions."Dequeue", "Error In"=w237) -> ("Error Out"=w229:errorcluster, "Message Packet [Out]"=w231:T24)  [unwired: 4 in, 3 out]
    n81 = Unbundle By Name(w231) -> ("Message"=w230:string)
    n82 = case shown="\"Process\"" w230 {
      tunnel: w229 -> [w238 w240 w245]
      tunnel: [w238 w240 w241] -> w228
      tunnel: [_ TRUE _] -> w227
      frame "Init", Default {
      }
      frame "Exit" {
      }
      frame "Process" {
        n83 = call "Data Queue.vi"("Action"=Queue_Manager_Actions."Dequeue", "error in (no error)"=w245) -> ("error out"=w244:errorcluster, "data out"=w242:sgl[])  [unwired: 7 in, 1 out]
        n84 = Empty Array?(array=w242) -> (empty?=w243:bool)
        n85 = case shown="False" w243 {
          tunnel: w244 -> [w255 w281]
          tunnel: [w248 w281] -> w241
          tunnel: w242 -> [w254 _]
          frame False {
            n86 = local read "Save?"() -> (w252:bool)
            n87 = case shown="True" w252 {
              tunnel: [w264 w275] -> w253
              tunnel: w255 -> [w264 w270]
              tunnel: w254 -> [_ w272]
              frame False {
              }
              frame True {
                n88 = call "System Parameters - FGV.vi"("Actions"=FGV_Actions."Get", "Error In"=w270) -> ("Error Out"=w268:errorcluster, "System Parameters"=w269:T26)  [unwired: 8 in]
                n89 = Unbundle By Name(w269) -> ("Imaging Parameter.Custom Size.X"=w265:u16)
                n90 = call "Data Trim Module.vi"("#pixels to save"="#pixels to save", "error in"=w268, "start pixel"="Start pixel for save", "#A-lines"=w265, "1D Array in"=w272) -> ("error out"=w274:errorcluster, "array for saving"=w273:sgl[])  [unwired: 5 in]
                n91 = call "Save Data Queue.vi"("Action"=Queue_Manager_Actions."Enqueue", "error in (no error)"=w274, "data in"=w273) -> ("error out"=w276:errorcluster)  [unwired: 5 in, 3 out]
                n92 = call "Queue Manager.vi"("Queue Name"=QueueNames."Main Saving", "Action"=Queue_Manager_Actions."Enqueue", "Error In"=w276, "Message Packet Array"=T24[] [{"Message"="Save", "Parameter"=variant}]) -> ("Error Out"=w275:errorcluster)  [unwired: 3 in, 4 out]
              }
            }
            n93 = disable-structure shown="Enabled" {
              disable-tunnel: w254 -> [w260 _]
              disable-tunnel: w253 -> [w258 w263]
              disable-tunnel: [w256 w263] -> w249
              frame Enabled {
                n94 = call "Display Queue.vi"("Action"=Queue_Manager_Actions."Flush Queue", "error in (no error)"=w258) -> ("error out"=w259:errorcluster)  [unwired: 5 in, 4 out]
                n95 = call "Display Queue.vi"("Action"=Queue_Manager_Actions."Enqueue", "error in (no error)"=w259, "time out"=5, "input data"=w260) -> ("error out"=w256:errorcluster)  [unwired: 3 in, 4 out]
              }
              frame Disabled {
              }
            }
            n96 = call "Queue Manager.vi"("Queue Name"=QueueNames."Main Display", "Action"=Queue_Manager_Actions."Enqueue", "Error In"=w249, "Message Packet Array"=T24[] [{"Message"="Update Image", "Parameter"=variant}]) -> ("Error Out"=w248:errorcluster)  [unwired: 3 in, 4 out]
          }
          frame True {
          }
        }
      }
    }
    n97 = call "Error Message Handler.vi"("Error In"=w228) -> ("Error Out"=w234:errorcluster, "T button?"=w232:bool)  [unwired: 9 in]
    n98 = case shown="False" w232 {
      tunnel: w234 -> [w282 w284]
      tunnel: [w282 w285] -> w233
      frame False {
      }
      frame True {
        n99 = call "Queue Manager.vi"("Queue Name"=QueueNames."Main Processing", "Action"=Queue_Manager_Actions."Enqueue", "Error In"=w284, "Message Packet Array"=T24[] [{"Message"="Exit", "Parameter"=variant}] ("Message Packet [In]")) -> ("Error Out"=w285:errorcluster)  [unwired: 3 in, 4 out]
      }
    }
  }
  n100 = while {
    shift-right: [w289] -> w9
    shift-left: w1 -> [w298]
    shift-right: [w300] -> _
    shift-left: _ -> [w299]
    stop <- w301 stop-if-true
    # "Main Display"
    n101 = call "Queue Manager.vi"("Queue Name"=QueueNames."Main Display", "Action"=Queue_Manager_Actions."Dequeue", "Error In"=w298) -> ("Error Out"=w295:errorcluster, "Message Packet [Out]"=w294:T24)  [unwired: 4 in, 3 out]
    n102 = Unbundle(w294) -> ("Message"=w293:string, "Parameter"=w292:variant)
    n103 = case shown="\"Update Image\"" w293 {
      tunnel: w295 -> [w312 w324 w338 w348 w350 w352]
      tunnel: w292 -> [_ _ _ _ _ _]
      tunnel: [w310 w315 w339 w347 w350 w352] -> w291
      tunnel: [TRUE _ _ _ _ _] -> w301
      tunnel: [_ w318 w343 w344 w349 w351] -> w300
      tunnel: w299 -> [_ _ w343 w344 w349 w351]
      frame "Exit", Default {
        n104 = call "RAW Image Buffer.vi"("Actions"=enum16{"Init", "Create", "Get", "Dispose"}."Dispose", "Error In"=w312) -> ("Error Out"=w311:errorcluster, "Image Out"=w308:T21)  [unwired: 8 in]
        n105 = local write "Image"(w308) -> ()
        n106 = call "Image Queue.vi"("Action"=Queue_Manager_Actions."Release Queue", "Error In"=w311) -> ("Error Out"=w310:errorcluster)  [unwired: 8 in, 1 out]
      }
      frame "Init" {
        w319 = T30 2 items=["Grayscale (U8)", "Grayscale (I16)", "Grayscale (SGL)", "Complex (CSG)", "RGB (U32)", "HSL (U32)", "RGB (U64)", "Grayscale (U16)"] ("Image Type")
        n107 = call "RAW Image Buffer.vi"("Actions"=enum16{"Init", "Create", "Get", "Dispose"}."Init", "Error In"=w324) -> ("Error Out"=w323:errorcluster)  [unwired: 8 in, 1 out]
        n108 = call "RAW Image Buffer.vi"("Actions"=enum16{"Init", "Create", "Get", "Dispose"}."Create", "Error In"=w323) -> ("Error Out"=w317:errorcluster)  [unwired: 8 in, 1 out]
        n109 = disable-structure shown="Enabled" {
          disable-tunnel: w317 -> [w326 w330]
          disable-tunnel: [w325 w330] -> w316
          frame Disabled {
            n110 = call "Queue Manager.vi"("Queue Name"=QueueNames."Main Display", "Action"=Queue_Manager_Actions."Enqueue", "Error In"=w326, "Message Packet Array"=T24[] [{"Message"="Update Image", "Parameter"=variant}]) -> ("Error Out"=w325:errorcluster)  [unwired: 3 in, 4 out]
          }
          frame Enabled {
          }
        }
        n111 = call "IMAQ Create"("Image Name"="test", "Image Type"=w319, "error in (no error)"=w316) -> ("New Image"=w318:T21, "error out"=w315:errorcluster)  [unwired: 2 in]
      }
      frame "Update Image" {
        w332 = u32 20  # acquire extra 25 A-lines to account for the DAQ frame trigger jitter
        n112 = call "System Parameters - FGV.vi"("Actions"=FGV_Actions."Get", "Error In"=w338) -> ("Error Out"=w337:errorcluster, "System Parameters"=w335:T26)  [unwired: 8 in]
        n113 = Unbundle By Name(w335) -> ("Imaging Parameter.Custom Size.X"=w333:u16)
        n114 = Wait (ms)(milliseconds to wait=u32 40) -> ()  [unwired: 1 out]
        n115 = Add(x=w332, y=w333) -> (x+y=w331:u32)
        n116 = call "Display_Module.vi"("Start pixel for display"="Start pixel for display", "FOV: #A-lines"=w331, "error in"=w337, "Total pixels to display"="#pixels to display", "Source in"=w343) -> ("error out"=w339:errorcluster, "Image"=→"Image":T21)  [unwired: 5 in]
      }
      frame "Update Status" {
        n117 = call "Status Queue.vi"("Action"=Queue_Manager_Actions."Get Status", "Error In"=w348) -> ("Error Out"=w347:errorcluster, "Status Message [Out]"=w345:string)  [unwired: 8 in]
        n118 = local write "Status"(w345) -> ()
      }
      frame "Update Line Profile" {
      }
      frame "Idle" {
      }
    }
    n119 = call "Error Message Handler.vi"("Error In"=w291) -> ("Error Out"=w290:errorcluster, "T button?"=w288:bool)  [unwired: 9 in]
    n120 = case shown="False" w288 {
      tunnel: [w302 w305] -> w289
      tunnel: w290 -> [w302 w303]
      frame False {
      }
      frame True {
        n121 = call "Queue Manager.vi"("Queue Name"=QueueNames."Main Display", "Action"=Queue_Manager_Actions."Enqueue", "Error In"=w303, "Message Packet Array"=T24[] [{"Message"="Exit", "Parameter"=variant}] ("Message Packet [In]")) -> ("Error Out"=w305:errorcluster)  [unwired: 3 in, 4 out]
      }
    }
  }
  n122 = while {
    shift-right: [w354] -> w16
    shift-left: w1 -> [w363]
    stop <- w364 stop-if-true
    # "Main GUI"
    n123 = call "Queue Manager.vi"("Queue Name"=QueueNames."Main GUI", "Action"=Queue_Manager_Actions."Dequeue", "Error In"=w363) -> ("Error Out"=w361:errorcluster, "Message Packet [Out]"=w360:T24)  [unwired: 4 in, 3 out]
    n124 = Unbundle(w360) -> ("Message"=w357:string, "Parameter"=w359:variant)
    n125 = case shown="\"Wait for User Input\"" w357 {
      tunnel: w361 -> [w379 w405 w416 w443 w450 w464 w476 w588 w591]
      tunnel: w359 -> [_ _ _ _ _ _ _ _ _]
      tunnel: [w378 w401 w412 w435 w446 w462 w477 w589 w591] -> w353
      tunnel: [_ _ _ _ _ _ _ TRUE _] -> w364
      frame "Init" {
        n126 = call "Queue Manager.vi"("Queue Name"=QueueNames."Main GUI", "Action"=Queue_Manager_Actions."Enqueue", "Error In"=w379, "Message Packet Array"=T24[] [{"Message"="Init Variables", "Parameter"=variant}, {"Message"="Set Front Panel", "Parameter"=variant}, {"Message"="Update User Settings", "Parameter"=variant}, {"Message"="Configure Hardware", "Parameter"=variant}, {"Message"="Wait for Complete", "Parameter"=variant}, {"Message"="Wait for User Input", "Parameter"=variant}]) -> ("Error Out"=w378:errorcluster)  [unwired: 3 in, 4 out]
      }
      frame "Init Variables" {
        w387 = Queue_Manager_Actions."Init" ("Action")
        (unwired) enum32{"Scan", "Config", "Manual Contorls"}."Scan" ("Control Panel")
        n127 = call "Status Queue.vi"("Action"=Queue_Manager_Actions."Enqueue", "Error In"=w405, "Status Message [In]"="Initializing Variables...") -> ("Error Out"=w400:errorcluster)  [unwired: 7 in, 1 out]
        n128 = control-ref of="This VI"() -> (w403:refnum<vi>)
        n129 = call "Defer Panel Updates.vi"("Action"=enum16{"Init", "Freeze", "Unfreeze"}."Init", "Error In"=w400, "reference"=w403) -> ("Error Out"=w384:errorcluster)  [unwired: 8 in]
        n130 = call "Image Queue.vi"("Action"=Queue_Manager_Actions."Init", "Error In"=w384) -> ("Error Out"=w381:errorcluster)  [unwired: 8 in, 1 out]
        n131 = call "System Parameters - FGV.vi"("Actions"=FGV_Actions."Init", "Error In"=w381) -> ("Error Out"=w391:errorcluster)  [unwired: 8 in, 1 out]
        n132 = call "Data Queue.vi"("max queue size (-1, unlimited)"=100 ("y"), "Action"=w387, "error in (no error)"=w391) -> ("error out"=w383:errorcluster)  [unwired: 6 in, 2 out]
        n133 = call "Display Queue.vi"("Action"=w387, "error in (no error)"=w383, "max queue size (-1, unlimited)"=100) -> ("error out"=w388:errorcluster)  [unwired: 4 in, 4 out]
        n134 = call "Save Data Queue.vi"("max queue size (-1, unlimited)"=100, "Action"=w387, "error in (no error)"=w388) -> ("error out"=w389:errorcluster)  [unwired: 5 in, 3 out]
        n135 = disable-structure shown="Enabled" {
          disable-tunnel: [w407 w411] -> w380
          disable-tunnel: w389 -> [w406 w411]
          frame Enabled {
            n136 = call "Read Config from File.vi"("error in (no error)"=w406) -> ("error out"=w410:errorcluster, "System Parameters"=w408:T26)  [unwired: 9 in]
            n137 = call "System Parameters - FGV.vi"("Actions"=FGV_Actions."Set", "Error In"=w410, "System Parameters [In]"=w408) -> ("Error Out"=w407:errorcluster)  [unwired: 7 in, 1 out]
          }
          frame Disabled {
          }
        }
        n138 = control-ref of="Imaging Parameter"() -> (w393:refnum<vi>)
        n139 = call "Set Front Panel Custom Image Size Cluster Control.vi"("error in (no error)"=w380, "Enable/Disable"=FALSE, "Init"=TRUE, "Imaging Parameter"=w393) -> ("error IO"=w395:errorcluster)  [unwired: 7 in]
        n140 = call "FGV - Acquisition Status.vi"("Actions"=FGV_Actions."Init", "Error In"=w395) -> ("Error Out"=w401:errorcluster, "Scan Type [Out]"=w396:T6)  [unwired: 5 in, 3 out]
        n141 = local write "Scan Type"(w396) -> ()
      }
      frame "Set Front Panel" {
        n142 = call "Status Queue.vi"("Action"=Queue_Manager_Actions."Enqueue", "Error In"=w416, "Status Message [In]"="Setting Front Panel Controls...") -> ("Error Out"=w417:errorcluster)  [unwired: 7 in, 1 out]
        n143 = call "Defer Panel Updates.vi"("Action"=enum16{"Init", "Freeze", "Unfreeze"}."Freeze", "Error In"=w417) -> ("Error Out"=w425:errorcluster)  [unwired: 9 in]
        n144 = call "FGV - Acquisition Status.vi"("Actions"=FGV_Actions."Get", "Error In"=w425) -> ("Error Out"=w422:errorcluster, "Scan Type [Out]"=w420:T6, "Level Status Out"=w421:bool)  [unwired: 5 in, 2 out]
        n145 = case "Acquiring?" shown="False" w421 {
          tunnel: [w429 w434] -> w423
          tunnel: w422 -> [w430 w434]
          tunnel: w420 -> [w428 _]
          frame False {
            # "Non-Acquiring FP States"
            n146 = disable-structure shown="Enabled" {
              disable-tunnel: w430 -> [w433 _]
              disable-tunnel: [w432 _] -> w429
              disable-tunnel: w428 -> [w431 _]
              frame Disabled {
                n147 = call "Set Main GUI for Different Acquire States.vi"("Error In"=w433, "Scan Type [Out]"=w431) -> ("Error Out"=w432:errorcluster)  [unwired: 9 in]
              }
              frame Enabled {
              }
            }
          }
          frame True {
            # "Acquiring FP States"
          }
        }
        n148 = call "Defer Panel Updates.vi"("Action"=enum16{"Init", "Freeze", "Unfreeze"}."Unfreeze", "Error In"=w423) -> ("Error Out"=w413:errorcluster)  [unwired: 9 in]
        n149 = call "Status Queue.vi"("Action"=Queue_Manager_Actions."Enqueue", "Error In"=w413, "Status Message [In]"="Finished Setting Front Panel.") -> ("Error Out"=w412:errorcluster)  [unwired: 7 in, 1 out]
      }
      frame "Update User Settings" {
        n150 = disable-structure shown="Enabled" {
          disable-tunnel: [_ Queue_Manager_Actions."Enqueue" ("Action")] -> w437
          frame Disabled {
            n151 = local read "Vibratome"() -> ()  [unwired: 1 in]
            n152 = local read "Imaging Parameter"() -> ()  [unwired: 1 in]
            n153 = local read "Optical Parameters"() -> ()  [unwired: 1 in]
          }
          frame Enabled {
          }
        }
        n154 = call "Status Queue.vi"("Action"=w437, "Error In"=w443, "Status Message [In]"="Loading User Settings...") -> ("Error Out"=w441:errorcluster)  [unwired: 7 in, 1 out]
        n155 = call "Defer Panel Updates.vi"("Action"=enum16{"Init", "Freeze", "Unfreeze"}."Freeze", "Error In"=w441) -> ("Error Out"=w436:errorcluster)  [unwired: 9 in]
        n156 = call "Set Front Panel Custom Image Size Cluster Control.vi"("error in (no error)"=w436, "Enable/Disable"=TRUE) -> ("error IO"=w439:errorcluster)  [unwired: 9 in]
        n157 = call "Defer Panel Updates.vi"("Action"=enum16{"Init", "Freeze", "Unfreeze"}."Unfreeze", "Error In"=w439) -> ("Error Out"=w435:errorcluster)  [unwired: 9 in]
      }
      frame "Configure Hardware" {
        n158 = call "Status Queue.vi"("Action"=Queue_Manager_Actions."Enqueue", "Error In"=w450, "Status Message [In]"="Initializing Hardware...") -> ("Error Out"=w449:errorcluster)  [unwired: 7 in, 1 out]
        n159 = Build Array(T24 {"Message"="Init Hardware", "Parameter"=variant} ("Message Packet [In]")) -> (w447:T24[])
        n160 = call "Queue Manager.vi"("Queue Name"=QueueNames."Main Scan Processor", "Action"=Queue_Manager_Actions."Enqueue", "Error In"=w449, "Message Packet Array"=w447) -> ("Error Out"=w446:errorcluster)  [unwired: 3 in, 4 out]
      }
      frame "Wait for Complete" {
        n161 = call "TickTock.vi"("Error In"=w464) -> ("Error Out"=w460:errorcluster, "Current Time (Out)"=w459:timestamp)  [unwired: 8 in, 1 out]
        n162 = while {
          shift-right: [w467] -> w461
          shift-left: w460 -> [w475]
          tunnel: w459 -> [w474]
          tunnel: [w465] -> w458
          stop <- w466 stop-if-true
          n163 = call "Inline Wait.vi"("Error In"=w475, "milliseconds to wait"=u32 100) -> ("Error Out"=w471:errorcluster)  [unwired: 9 in]
          n164 = call "TickTock.vi"("Error In"=w471, "Current Time (In)"=w474) -> ("Error Out"=w467:errorcluster, "dt"=w473:dbl)  [unwired: 7 in, 1 out]
          n165 = Greater?(x=60000.0, y=w473) -> (0:w465:bool)
          n166 = global read "Main Scan Processor Status.vi" "Busy"() -> (w469:bool)
          n167 = Not(x=w469) -> (.not. x?=w468:bool)
          n168 = Or(x=w465, y=w468) -> (x .or. y?=w466:bool)
        }
        n169 = Select(t="Completed." ("Status Message [In]"), s=w458, f="Operation timed out." ("Status Message [In]")) -> (s? t:f=w455:string)
        n170 = call "Status Queue.vi"("Action"=Queue_Manager_Actions."Enqueue", "Error In"=w461, "Status Message [In]"=w455) -> ("Error Out"=w462:errorcluster)  [unwired: 7 in, 1 out]
      }
      frame "Wait for User Input" {
        n171 = event shown="[6] \"Acquire\": Value Change" {
          selector: _ -> [_ _ _ _ _ _ _]
          dyn-events: _ -> [_ _ _ _ _ _ _]
          timeout: _ -> [_ _ _ _ _ _ _]
          tunnel: [w478 w495 w501 w517 w530 w543 w562] -> w477
          tunnel: w476 -> [w478 w483 w503 w514 w534 w539 w563]
          event Timeout {
            n172 = event-data() -> ()  [unwired: 1 in, 3 out]
          }
          event "Quit": Value Change {
            n173 = event-data() -> ()  [unwired: 1 in, 1 out]
            n174 = call "FGV - Acquisition Status.vi"("Actions"=FGV_Actions."Get", "Error In"=w483) -> ("Error Out"=w482:errorcluster, "Scan Type [Out]"=w480:T6)  [unwired: 5 in, 3 out]
            n175 = call "FGV - Acquisition Status.vi"("Actions"=FGV_Actions."Set", "Error In"=w482, "Scan Type [In]"=w480, "Level Status In"=FALSE ("Status In")) -> ("Error Out"=w481:errorcluster)  [unwired: 3 in, 4 out]
            n176 = call "Queue Manager.vi"("Action"=Queue_Manager_Actions."Flush All Queues", "Error In"=w481) -> ("Error Out"=w486:errorcluster)  [unwired: 5 in, 4 out]
            n177 = call "Status Queue.vi"("Action"=Queue_Manager_Actions."Enqueue", "Error In"=w486, "Status Message [In]"="Exiting Software...") -> ("Error Out"=w491:errorcluster)  [unwired: 7 in, 1 out]
            n178 = call "Set Main GUI for Different Acquire States.vi"("Error In"=w491, "Scan Type [Out]"=ScanType."Single Frame") -> ("Error Out"=w490:errorcluster)  [unwired: 9 in]
            n179 = call "Queue Manager.vi"("Action"=Queue_Manager_Actions."Enqueue All", "Error In"=w490, "Message Packet Array"=T24[] [{"Message"="Exit", "Parameter"=variant}] ("Message Packet [In]")) -> ("Error Out"=w495:errorcluster)  [unwired: 4 in, 4 out]
          }
          event "Image": Value Change {
            w504 = 2 items=["No Event"=0, "Click Event"=1, "Draw Event"=2, "Size Event"=4, "Scroll Event"=5, "Double Click Event"=8]
            n180 = event-data() -> ("CtlRef"=w496:refnum<vi>)  [unwired: 1 in, 5 out]
            n181 = Build Array(w504) -> (w505:i32[])
            n182 = invoke class="ImageControl" method="Get Last Event"(reference=w496, error in=w503, "Which Events"=w505) -> (error out=w502:errorcluster)  [unwired: 5 in, 7 out]
            n183 = Build Array(T24 {"Message"="Wait for User Input", "Parameter"=variant} ("Message Packet [In]")) -> (w497:T24[])
            n184 = call "Queue Manager.vi"("Queue Name"=QueueNames."Main GUI", "Action"=Queue_Manager_Actions."Enqueue", "Error In"=w502, "Message Packet Array"=w497) -> ("Error Out"=w501:errorcluster)  [unwired: 3 in, 4 out]
          }
          event Value Change {
            n185 = event-data() -> ("NewVal"=w509:T31)  [unwired: 1 in]
            n186 = Add(x=w509, y=5) -> (x+y=w523:i32)
            n187 = Power Of 2(x=w523) -> (2^x=w522:dbl)
            n188 = call "System Parameters - FGV.vi"("Actions"=FGV_Actions."Get", "Error In"=w514) -> ("Error Out"=w513:errorcluster, "System Parameters"=w511:T26)  [unwired: 8 in]
            n189 = Bundle By Name(cluster=w511, "Imaging Parameter.XY Image Size"=w509) -> (w510:T26)
            n190 = local read "Imaging Parameter"() -> (w508:T4)
            n191 = To Unsigned Word Integer(number=w522) -> (unsigned 16bit integer=w506:u16)
            n192 = Bundle By Name(cluster=w508, "Custom Size.X"=w506, "Custom Size.Y"=w506) -> (w507:T4)
            n193 = local write "Imaging Parameter"(w507) -> ()
            n194 = call "System Parameters - FGV.vi"("Actions"=FGV_Actions."Set", "Error In"=w513, "System Parameters [In]"=w510) -> ("Error Out"=w512:errorcluster)  [unwired: 7 in, 1 out]
            n195 = Build Array(T24 {"Message"="Wait for User Input", "Parameter"=variant} ("Message Packet [In]")) -> (w518:T24[])
            n196 = call "Queue Manager.vi"("Queue Name"=QueueNames."Main GUI", "Action"=Queue_Manager_Actions."Enqueue", "Error In"=w512, "Message Packet Array"=w518) -> ("Error Out"=w517:errorcluster)  [unwired: 3 in, 4 out]
          }
          event Value Change {
            n197 = event-data() -> ()  [unwired: 1 in, 6 out]
            n198 = call "FGV - Acquisition Status.vi"("Actions"=FGV_Actions."Get") -> ("Level Status Out"=w529:bool)  [unwired: 6 in, 4 out]
            n199 = call "FGV - Acquisition Status.vi"("Actions"=FGV_Actions."Set", "Hardware in"="Hardware in", "Scan Type [In]"="Scan Type", "Level Status In"=w529) -> ()  [unwired: 3 in, 5 out]
            n200 = call "Queue Manager.vi"("Queue Name"=QueueNames."Main GUI", "Action"=Queue_Manager_Actions."Enqueue", "Error In"=w534, "Message Packet Array"=T24[] [{"Message"="Set Front Panel", "Parameter"=variant}, {"Message"="Wait for User Input", "Parameter"=variant}]) -> ("Error Out"=w530:errorcluster)  [unwired: 3 in, 4 out]
          }
          event "Save?": Value Change {
            n201 = event-data() -> ()  [unwired: 1 in, 6 out]
            n202 = call "Queue Manager.vi"("Queue Name"=QueueNames."Main GUI", "Action"=Queue_Manager_Actions."Enqueue", "Error In"=w539, "Message Packet Array"=T24[] [{"Message"="Wait for User Input", "Parameter"=variant}]) -> ("Error Out"=w536:errorcluster)  [unwired: 3 in, 4 out]
            n203 = call "FGV - Acquisition Status.vi"("Actions"=FGV_Actions."Get", "Error In"=w536) -> ("Error Out"=w537:errorcluster, "Scan Type [Out]"=w535:T6)  [unwired: 5 in, 3 out]
            n204 = case shown="\"Single Frame\", Default" w535 {
              tunnel: [w544 w549] -> w543
              tunnel: w537 -> [w544 w545]
              frame "Single Frame", Default {
              }
              frame "Mosaic" {
                n205 = local read "path"() -> (w548:path)
                n206 = call "Write Mosaic Positions.vi"("path"=w548) -> ("appended path"=w546:path)  [unwired: 10 in]
                n207 = call "Save as Text2.vi"("action"="Open", "error in"=w545, "file path (use dialog)"=w546) -> ("error out"=w549:errorcluster)  [unwired: 8 in]
              }
            }
          }
          event "Acquire": Value Change {
            w561 = Queue_Manager_Actions."Enqueue" ("Action")
            n208 = event-data() -> ()  [unwired: 1 in, 6 out]
            n209 = call "Queue Manager.vi"("Queue Name"=QueueNames."Main GUI", "Action"=w561, "Error In"=w563, "Message Packet Array"=T24[] [{"Message"="Wait for User Input", "Parameter"=variant}]) -> ("Error Out"=w552:errorcluster)  [unwired: 3 in, 4 out]
            n210 = call "FGV - Acquisition Status.vi"("Actions"=FGV_Actions."Get", "Error In"=w552) -> ("Error Out"=w553:errorcluster, "Hardware out"=w551:T7, "Scan Type [Out]"=w554:T6, "Level Status Out"=w555:bool)  [unwired: 5 in, 1 out]
            n211 = case "Start Acquisition?" shown="False" w555 {
              tunnel: w552 -> [w579 w584]
              tunnel: [w583 w584] -> w562
              tunnel: w561 -> [w582 _]
              frame False {
                # "Starts Acquisition if Current Acquisition Status is \"Off\""
                n212 = Unbundle By Name("Imaging Parameter") -> ("Custom Size.Y"=w568:u16)
                n213 = Add(x=w568, y=u16 20) -> (x+y=w567:u16)
                n214 = Bundle By Name(cluster="Alazar parameters", "Acq Settings.Records Per Buffer"=w567) -> (w569:T8)
                n215 = Bundle By Name(cluster=T26 {"Optical Parameters"={"Obj. Focal Length [mm]"=0.0, "Scan Lens EFL[mm]"=0.0, "Tube Lens EFL[mm]"=0.0, "Galvo V Range (+/-)"=0.0, "Galvo Max Half Angle [Deg]"=0.0, "Max Galvo Range[%]"=0.0}, "Vibratome"={"Z Bottom [mm]"=0.0, "Pre Cut Dwell [s]"=0.0, "Blade Frequency [RPM]"=0, "Slice Speed [mm/s]"=0.0, "Post Cut Dwell [s]"=0.0, "Ramp Time [s]"=0.0, "Start X [mm]"=0.0, "Start Y [mm]"=0.0, "Slice Length [mm]"=0.0, "Slice Axis"=enum."Y Axis", "Controller VISA Ref"="COM4"}, "Table Stages"={"X Stage"={"Position"=0.0, "Is.Enabled?"=FALSE, "Is.Connected?"=FALSE, "Device SN"="45876539", "AccelerationMaximum"=0.0, "VelocityMaximum"=0.0, "Acceleration"=0.0, "Velocity"=0.0, "waitTimeout (ms)"=0, "Model"=enum."None", "Is.Homed?"=FALSE}, "Y Stage"={"Position"=0.0, "Is.Enabled?"=FALSE, "Is.Connected?"=FALSE, "Device SN"="45876539", "AccelerationMaximum"=0.0, "VelocityMaximum"=0.0, "Acceleration"=0.0, "Velocity"=0.0, "waitTimeout (ms)"=0, "Model"=enum."None", "Is.Homed?"=FALSE}, "Z Stage"={"Position"=0.0, "Is.Enabled?"=FALSE, "Is.Connected?"=FALSE, "Device SN"="45876539", "AccelerationMaximum"=0.0, "VelocityMaximum"=0.0, "Acceleration"=0.0, "Velocity"=0.0, "waitTimeout (ms)"=0, "Model"=enum."None", "Is.Homed?"=FALSE}}, "Imaging Parameter"={"Raster Scan Direction"=enum."Bi Directional", "Pixel Dwell Time [Clock Cycles]"=1, "Flyback Time [Clock Cycles]"=0, "XY Center [um]"={"X"=1.0, "Y"=1.0}, "Pixel Step Size [um]"=1.0, "XY Image Size"=enum."256 x 256", "Custom"=FALSE, "Custom Size"={"X"=1, "Y"=1}, "Line Averages"=1}, "Galvo HW Parameters"={"Analog Out Channel"="GalvoCtrl/ao0,GalvoCtrl/ao1", "Min Voltage"=-10.0, "Max Voltage"=10.0, "Pixel Clock Source"="/GalvoCtrl/PFI0", "Sample Rate"=1000.0, "Line Clock Out Ch"="GalvoCtrl/port0/line0"}, "Alazar parameters"={"Trigger Settings"={"General Trigger Settings"={"Trigger Operation"=0, "Coupling ID"=2, "Range ID"=2, "Delay"=0, "Timeout Ticks"=0, "Mode"=1, "Parameter"=1}, "Trigger Engine 1"={"Trigger Engine"=0, "Source"=2, "Slope"=1, "Level"=140}, "Trigger Engine 2"={"Trigger Engine"=1000, "Source"=4294967295, "Slope"=1, "Level"=2048}}, "Capture Clock"={"Sample Rate"=100, "Decimation"=0, "Source"=2, "Edge"=0}, "Device ID"={"System ID"=1, "Board ID"=1}, "Ch A Input Control"={"Channel"=1, "Coupling"=2, "Range"=10, "Impedance"=2}, "Ch B Input Control"={"Channel"=2, "Coupling"=2, "Range"=10, "Impedance"=2}, "Acq Settings"={"Window Type"=1, "Record Length"=1440, "Footer"=0, "Offset"=0, "Records Per Buffer"=2048, "Samples per record"=2048, "Records Count (Records/Acq)"=2147483647, "Output Format"=10}}, "Mosaic Paramter"={"X Axis"={"Start [mm]"=0.0, "Steps [pts]"=0, "End [mm]"=0.0}, "Y Axis"={"Start [mm]"=0.0, "Steps [pts]"=0, "End [mm]"=0.0}, "Scan Pattern"=enum."Uni-directional", "Overlap Options"={"Overlap Type"=enum."No Overlap", "Percent Overlap"=0, "Justify"=enum."Start"}}} ("System Parameters"), "Vibratome"="Vibratome", "Optical Parameters"="Optical Parameters", "Imaging Parameter"="Imaging Parameter", "Galvo HW Parameters"="Galvo HW Parameters", "Alazar parameters"=w569, "Table Stages"="Table Stages", "Mosaic Paramter"="Mosaic Paramter") -> (w564:T26)
                n216 = call "System Parameters - FGV.vi"("Actions"=FGV_Actions."Set", "Error In"=w579, "System Parameters [In]"=w564) -> ("Error Out"=w578:errorcluster)  [unwired: 7 in, 1 out]
                n217 = call "Queue Manager.vi"("Queue Name"=QueueNames."Main Scan Processor", "Action"=w582, "Error In"=w578, "Message Packet Array"=T24[] [{"Message"="Acquire", "Parameter"=variant}] ("Message Packet [In]")) -> ("Error Out"=w583:errorcluster)  [unwired: 3 in, 4 out]
              }
              frame True {
                # "Stops Acquisition if Current Status is On"
              }
            }
            n218 = Not(x=w555) -> (.not. x?=w556:bool)
            n219 = call "FGV - Acquisition Status.vi"("Edge Status In"=TRUE, "Actions"=FGV_Actions."Set", "Error In"=w553, "Hardware in"=w551, "Scan Type [In]"=w554, "Level Status In"=w556) -> ()  [unwired: 1 in, 5 out]
          }
        }
      }
      frame "Exit" {
        n220 = call "System Parameters - FGV.vi"("Actions"=FGV_Actions."Get", "Error In"=w588) -> ("Error Out"=w587:errorcluster, "System Parameters"=w585:T26)  [unwired: 8 in]
        n221 = call "Write Config to File.vi"("error in (no error)"=w587, "System Parameters"=w585) -> ("error out"=w589:errorcluster)  [unwired: 9 in]
      }
      frame Default {
      }
    }
    n222 = call "Error Message Handler.vi"("Error In"=w353) -> ("Error Out"=w356:errorcluster, "T button?"=w355:bool)  [unwired: 9 in]
    n223 = case shown="True" w355 {
      tunnel: w356 -> [w365 w366]
      tunnel: [w365 w367] -> w354
      frame False {
      }
      frame True {
        n224 = call "Status Queue.vi"("Action"=Queue_Manager_Actions."Enqueue", "Error In"=w366, "Status Message [In]"="Exiting Software...") -> ("Error Out"=w371:errorcluster)  [unwired: 7 in, 1 out]
        n225 = call "Set Main GUI for Different Acquire States.vi"("Error In"=w371, "Scan Type [Out]"=ScanType."Single Frame") -> ("Error Out"=w370:errorcluster)  [unwired: 9 in]
        n226 = call "Queue Manager.vi"("Action"=Queue_Manager_Actions."Enqueue All", "Error In"=w370, "Message Packet Array"=T24[] [{"Message"="Exit", "Parameter"=variant}] ("Message Packet [In]")) -> ("Error Out"=w367:errorcluster)  [unwired: 4 in, 4 out]
      }
    }
  }
  n227 = call "Queue Manager.vi"("Queue Name"=QueueNames."Main Display", "Action"=Queue_Manager_Actions."Release Queue", "Error In"=w9) -> ()  [unwired: 4 in, 5 out]
  n228 = call "Queue Manager.vi"("Queue Name"=QueueNames."Main Saving", "Action"=Queue_Manager_Actions."Release Queue", "Error In"=w5) -> ()  [unwired: 4 in, 5 out]
  n229 = call "Queue Manager.vi"("Queue Name"=QueueNames."Main Processing", "Action"=Queue_Manager_Actions."Release Queue", "Error In"=w2) -> ()  [unwired: 4 in, 5 out]
  n230 = call "Queue Manager.vi"("Queue Name"=QueueNames."Main Scan Processor", "Action"=Queue_Manager_Actions."Release Queue", "Error In"=w11) -> ()  [unwired: 4 in, 5 out]
  n231 = call "Queue Manager.vi"("Queue Name"=QueueNames."Main GUI", "Action"=Queue_Manager_Actions."Release Queue", "Error In"=w16) -> ()  [unwired: 4 in, 5 out]
